vi "Checkbarcode2.vi"(10 "String In":string="123456789\u0003") -> (2 "Complete":bool)   [LabVIEW 2014]
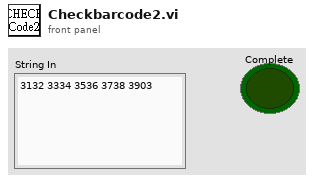
[diagram p1: front panel]
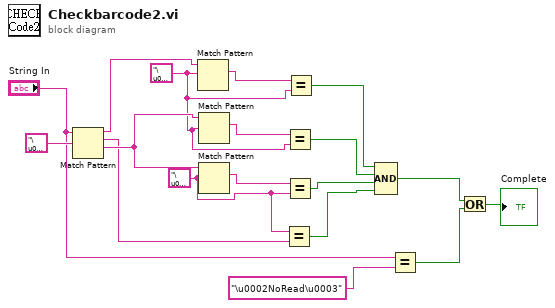
[diagram p0: block diagram]
diagram:
  w9 = "\u0002" ("regular expression")
  w13 = "\u0003" ("regular expression")
  n1 = Match Pattern(string="String In", regular expression="\u0003") -> (before substring=w6:string, match substring=w14:string, after substring=w15:string)  [unwired: 1 in, 1 out]
  n2 = Match Pattern(string=w6, regular expression=w9) -> (match substring=w8:string)  [unwired: 1 in, 3 out]
  n3 = Match Pattern(string=w15, regular expression=w9) -> (match substring=w18:string)  [unwired: 1 in, 3 out]
  n4 = Match Pattern(string=w15, regular expression=w13) -> (match substring=w17:string)  [unwired: 1 in, 3 out]
  n5 = Equal?(x=w13, y=w14) -> (x = y?=w10:bool)
  n6 = Equal?(x=w18, y=w9) -> (x = y?=w12:bool)
  n7 = Equal?(x=w17, y=w13) -> (x = y?=w11:bool)
  n8 = Equal?(x=w8, y=w9) -> (x = y?=w7:bool)
  n9 = Compound Arithmetic op=AND(w7, w12, w11, w10) -> (w3:bool)
  n10 = Equal?(x="String In", y="\u0002NoRead\u0003") -> (x = y?=w2:bool)
  n11 = Or(x=w3, y=w2) -> (x .or. y?=→"Complete":bool)
